vi "enes_suleyman_ozkan_170520517.vi"() -> ()   [LabVIEW 2020]
panel:
  out "KAPI AÇILDI":bool
  in  "ACÝL STOP":bool
  out "MESAFE":string
  out "return count":u32
  in  "byte count":u32
  in  "VISA resource name":refnum<visa-resource-name>
  # "VERÝ \nGÝRÝÞÝ"
  # "ENES ELEKTRONÝK A.Þ."
  # "GÜVENLÝK"
  # "MERKEZ"
  # "KAPI AÇILIYOR"
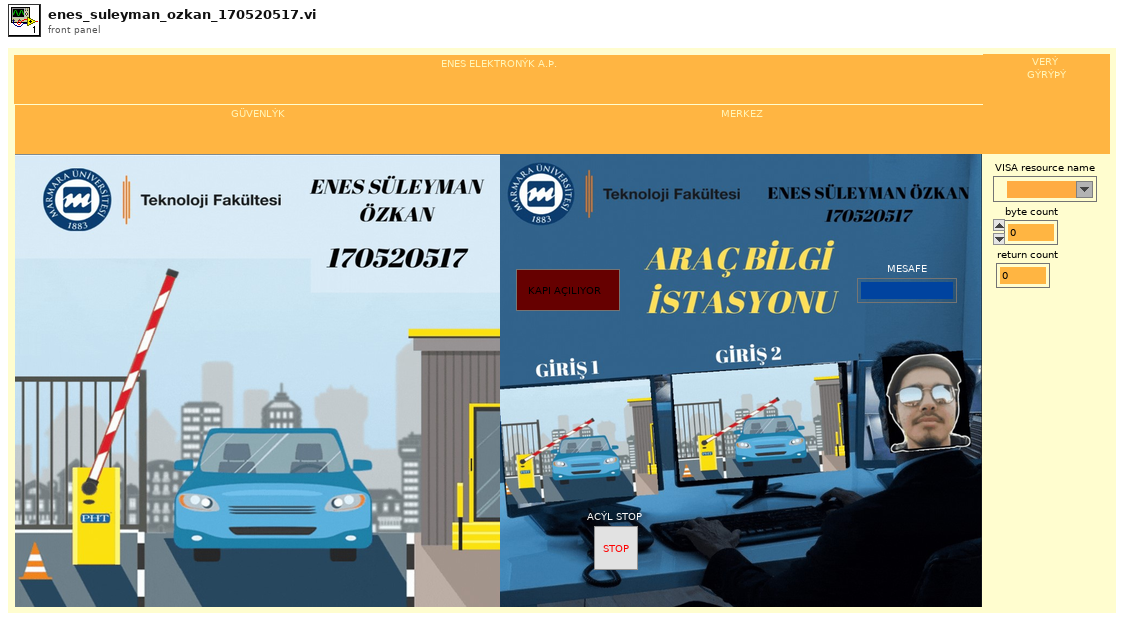
[diagram p1: front panel]
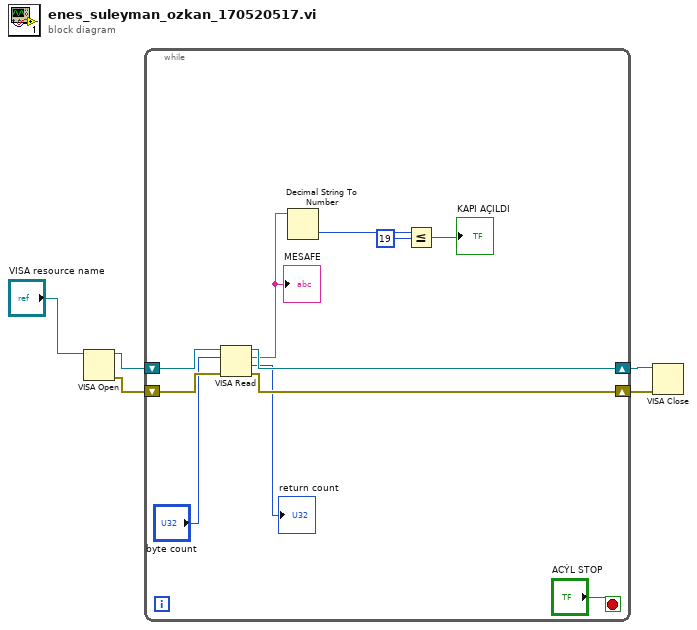
[diagram p0: block diagram]
diagram:
  n1 = VISA Open(VISA resource name="VISA resource name") -> (VISA resource name=w3:refnum<visa-resource-name>, error out=w4:errorcluster)  [unwired: 4 in]
  n2 = while {
    shift-right: [w14] -> w2
    shift-left: w4 -> [w16]
    shift-right: [w13] -> w1
    shift-left: w3 -> [w15]
    stop <- "ACÝL STOP" stop-if-true
    n3 = VISA Read(VISA resource name=w15, byte count="byte count", error in (no error)=w16) -> (VISA resource name out=w13:refnum<visa-resource-name>, read buffer=w9:string, return count=→"return count":u32, error out=w14:errorcluster)
    "MESAFE" <- w9
    n4 = Decimal String To Number(string=w9) -> (number=w7:i32)  [unwired: 2 in, 1 out]
    n5 = Less Or Equal?(x=w7, y=19) -> (x <= y?=→"KAPI AÇILDI":bool)
  }
  n6 = VISA Close(VISA resource name=w1, error in (no error)=w2) -> ()  [unwired: 1 out]
